vi "Config_Frequency.vi"(0 "reference in":refnum<class "DMM_Keysight_34980A.lvclass">, 5 "Voltage Range (5:Auto)":T3(ring)=enum."Auto", 7 "Low Frequency (1:20 Hz)":T2(ring)=enum."20 Hz", 9 "Aperture (1:100 ms)":T1(ring)=enum."100 ms", 11 "error in (no error)":errorcluster) -> (4 "reference in":refnum<class "DMM_Keysight_34980A.lvclass">, 15 "error out":errorcluster)   [LabVIEW 2022 SP3, in "DMM_Keysight_34980A.lvlib" / "DMM_Keysight_34980A.lvclass"]
uses:
  DMM_Keysight_34980A.lvclass
  Mode.ctl
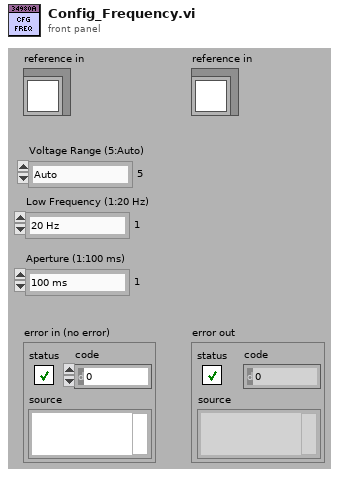
[diagram p1: front panel]
types:
  T1 = enum16{"10 ms", "100 ms", "1 sec", "Minimum", "Maximum"}
  T2 = enum16{"3 Hz", "20 Hz", "200 Hz", "Minimum", "Maximum"}
  T3 = enum16{"100 mV", "1 V", "10 V", "100 V", "300 V", "Auto", "Minimum", "Maximum"}
  T4 = typedef "DMM_Keysight_34980A.lvlib/DMM_Keysight_34980A.lvclass/Mode.ctl" = enum16{"DCV", "ACV", "2W Ohms", "4W Ohms", "Frequency", "DCA", "ACA"}
  T5 = typedef "DMM_Keysight_34980A.lvlib/DMM_Keysight_34980A.lvclass/ObjectAttributes.ctl" = cluster{"Config":T6, "VISA ref":refnum<visa-resource-name>, "Meas":dbl, "Range DCV":enum16{"100 mV", "1 V", "10 V", "100 V", "300 V", "Auto", "Minimum", "Maximum"}, "Range ACV":enum16{"100 mV", "1 V", "10 V", "100 V", "300 V", "Auto", "Minimum", "Maximum", "Default"}, "Range Ohms":enum16{"100 Ohm", "1 kOhm", "10 kOhm", "100 kOhm", "1 MOhm", "10 MOhm", "100 MOhm", "Auto", "Minimum", "Maximum"}, "Range VFreq":enum16{"100 mV", "1 V", "10 V", "100 V", "300 V", "Auto", "Minimum", "Maximum"}, " Range ACA":enum16{"10 mA", "100 mA", "1 A", "Auto", "Minimum", "Maximum"}, " Range DCA":enum16{"10 mA", "100 mA", "1 A", "Auto", "Minimum", "Maximum"}, "Mode":T4, "Resolution":enum16{"4 1/2", "5 1/2", "6 1/2", "Least", "Highest", "Default"}, "Bandwidth":enum16{"3 Hz", "20 Hz", "200 Hz", "Minimum", "Maximum"}, "Low Frequency":enum16{"3 Hz", "20 Hz", "200 Hz", "Minimum", "Maximum"}, "Aperture":enum16{"10 ms", "100 ms", "1 sec", "Minimum", "Maximum"}, "Measurement":dbl[], "Time":dbl[], "Samples":u32, "dt":dbl, "Timeout":dbl}
  T6 = typedef "DMM_Keysight_34980A.lvlib/DMM_Keysight_34980A.lvclass/Config.ctl" = cluster{"VISA":refnum<visa-resource-name>}
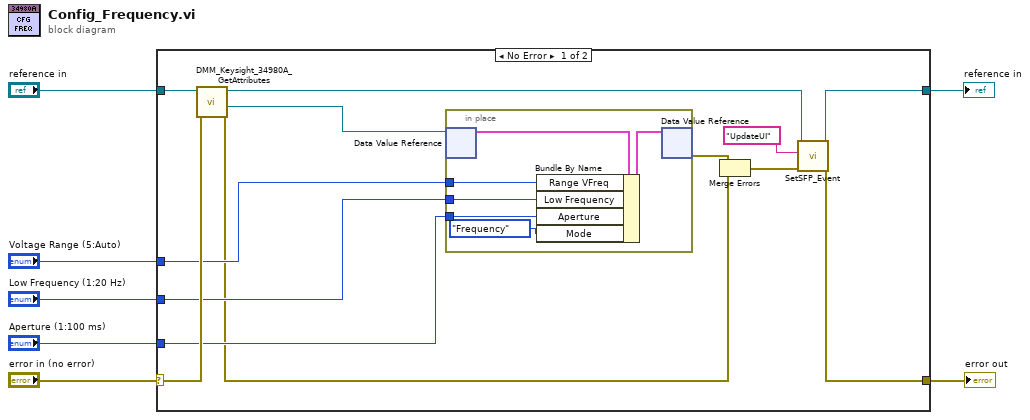
[diagram p0: block diagram]
diagram:
  n1 = case shown="No Error" "error in (no error)" {
    selector: "error in (no error)" -> [w20 w28]
    tunnel: [w15 w28] -> w6
    tunnel: [w16 w27] -> w4
    tunnel: "reference in" -> [w19 w27]
    tunnel: "Voltage Range (5:Auto)" -> [w11 _]
    tunnel: "Low Frequency (1:20 Hz)" -> [w10 _]
    tunnel: "Aperture (1:100 ms)" -> [w9 _]
    frame No Error {
      n2 = call "DMM_Keysight_34980A_GetAttributes.vi"("error in (no error)"=w20, "reference in"=w19) -> ("error out"=w8:errorcluster, "DataRef"=w18:refnum<data-value>, "reference out"=w17:refnum<class "DMM_Keysight_34980A.lvclass">)  [unwired: 6 in, 1 out]
      n3 = in-place {
        in-place-border: w11 -> [w24]
        in-place-border: w10 -> [w23]
        in-place-border: w9 -> [w22]
        n4 = in-place-dvr #1(w18) -> (w26:T5)  [unwired: 1 out]
        n5 = Bundle By Name(cluster=w26, "Range VFreq"=w24, "Low Frequency"=w23, "Aperture"=w22, "Mode"=Mode."Frequency") -> (w25:T5)
        n6 = in-place-dvr #1(w25) -> (w14:errorcluster)  [unwired: 1 out]
      }
      n7 = Merge Errors(w14, w8) -> (w13:errorcluster)
      n8 = call-dynamic "SetSFP_Event.vi"("error in (no error)"=w13, "msg"="UpdateUI", "reference in"=w17) -> ("error out"=w15:errorcluster, "reference out"=w16:refnum<class "DMM_Keysight_34980A.lvclass">)  [unwired: 7 in]
    }
    frame Error {
    }
  }
  "error out" <- w6
  "reference in" <- w4
